vi "RebootLogTimeFormat.vi"() -> (3 "time format":string="%Y-%m-%d %H:%M:%S")   [LabVIEW 2017, in "Controller.lvlib"]
uses:
  <vilib>/addons/InsightCM/Devices/Shared/Common/Controller/Controller.lvlib
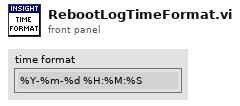
[diagram p1: front panel]
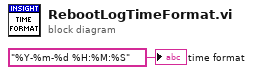
[diagram p0: block diagram]
diagram:
  "time format" <- "%Y-%m-%d %H:%M:%S" ("time format string (%c)")
